vi "apply mapping changes.vi"(4 "original channel":refnum<class "TBM channel.lvclass">, 6 "original tag":string, 7 "owner ID":string, 8 "error in":errorcluster, 9 "channel":refnum<class "TBM channel.lvclass">, 10 "tag name":string, 11 "engine configuration in":refnum<class "engine configuration.lvclass">) -> (0 "error out":errorcluster, 3 "engine configuration out":refnum<class "engine configuration.lvclass">)   [LabVIEW 2014, in "engine configuration.lvclass"]
doc: "This function is meant as a catch-all for any changes in a channel or in a tag. The function will look at the original tag and original channel, compare that to the new tag and new channel, and take any steps necessary to update the engine configuration appropriately."
uses:
  engine configuration.lvclass
  <vilib>/NI/Tag Bus Module Framework/channel/TBM channel.lvclass
  <vilib>/NI/Tag Bus/tag/tag descriptor.lvclass/tag descriptor.ctl
  <vilib>/NI/Tag Bus Module Framework/channel/TBM channel.lvclass/TBM channel.ctl
  <vilib>/NI/Tag Bus/tag/tag descriptor.lvclass
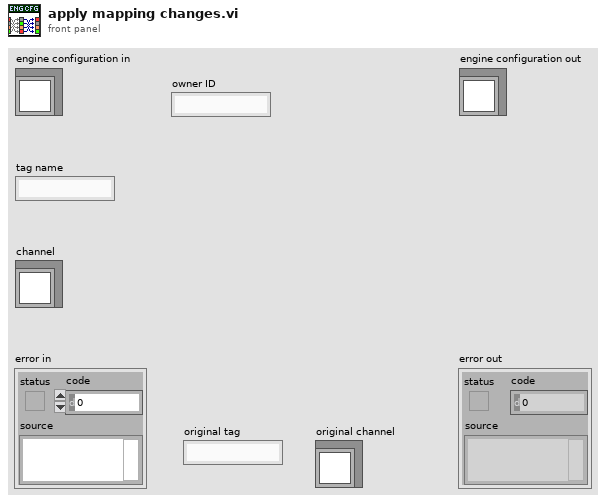
[diagram p1: front panel]
types:
  T1 = typedef "TBM channel.lvclass/channel classification.ctl" = enum16{"input data", "output data", "processing parameter", "processing result"}
  T2 = typedef "tag bus.lvlib/tag descriptor.lvclass/Data Type.ctl" = enum16{"Double", "Single", "I64", "I32", "I16", "I8", "U64", "U32", "U16", "U8", "Boolean", "String", "Array of Double", "Array of Single", "Array of I64", "Array of I32", "Array of I16", "Array of I8", "Array of U64", "Array of U32", "Array of U16", "Array of U8", "Array of Boolean", "Array of String"}
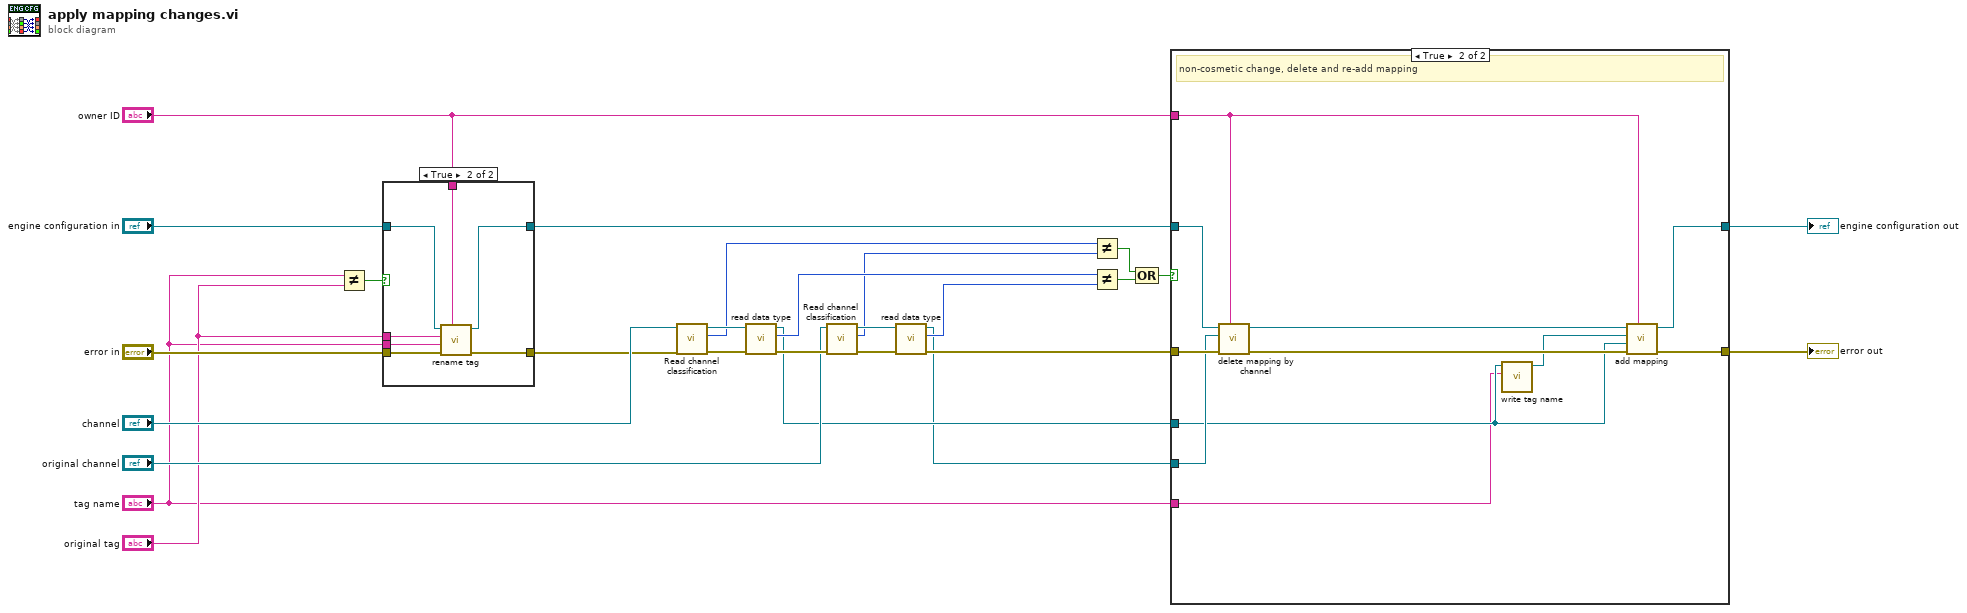
[diagram p0: block diagram]
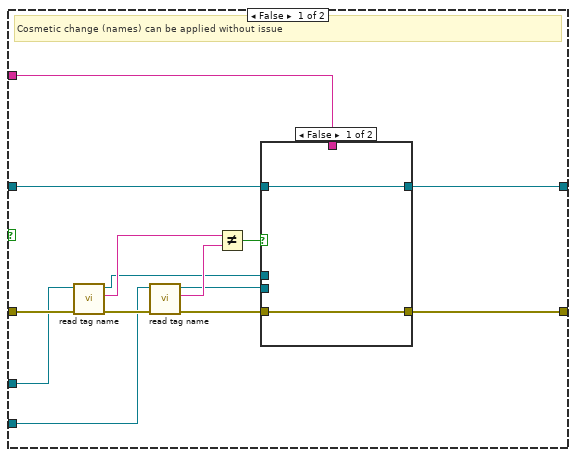
[diagram p3: hidden frame]
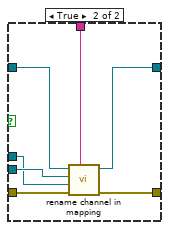
[diagram p4: hidden frame]
diagram:
  n1 = Not Equal?(x="tag name", y="original tag") -> (x != y?=w8:bool)
  n2 = case shown="True" w8 {
    tunnel: "error in" -> [w29 w36]
    tunnel: [w28 w34] -> w6
    tunnel: [w29 w35] -> w5
    tunnel: "engine configuration in" -> [w28 w33]
    tunnel: "owner ID" -> [_ w32]
    tunnel: "original tag" -> [_ w31]
    tunnel: "tag name" -> [_ w30]
    frame False {
    }
    frame True {
      n3 = call "rename tag.vi"("owner ID"=w32, "error in"=w36, "new name"=w30, "old name"=w31, "engine configuration in"=w33) -> ("error out"=w35:errorcluster, "engine configuration out"=w34:refnum<class "engine configuration.lvclass">)  [unwired: 5 in]
    }
  }
  n4 = call <vilib>:"Read channel classification.vi"("error in"=w5, "channel in"="channel") -> ("error out"=w25:errorcluster, "channel classification"=w14:T1, "channel out"=w26:refnum<class "TBM channel.lvclass">)  [unwired: 7 in]
  n5 = call <vilib>:"read data type.vi"("error in"=w25, "system tag in"=w26) -> ("error out"=w22:errorcluster, "data type"=w16:T2, "system tag out"=w12:refnum<class "TBM channel.lvclass">)  [unwired: 7 in]
  n6 = call <vilib>:"Read channel classification.vi"("error in"=w22, "channel in"="original channel") -> ("error out"=w24:errorcluster, "channel classification"=w15:T1, "channel out"=w23:refnum<class "TBM channel.lvclass">)  [unwired: 7 in]
  n7 = call <vilib>:"read data type.vi"("error in"=w24, "system tag in"=w23) -> ("error out"=w20:errorcluster, "data type"=w17:T2, "system tag out"=w11:refnum<class "TBM channel.lvclass">)  [unwired: 7 in]
  n8 = Not Equal?(x=w14, y=w15) -> (x != y?=w18:bool)
  n9 = Not Equal?(x=w16, y=w17) -> (x != y?=w19:bool)
  n10 = Compound Arithmetic op=OR(w18, w19) -> (w13:bool)
  n11 = case shown="True" w13 {
    tunnel: w20 -> [w41 w70]
    tunnel: w12 -> [w38 w61]
    tunnel: w11 -> [w37 w68]
    tunnel: w6 -> [w39 w69]
    tunnel: [w43 w65] -> w10
    tunnel: [w42 w64] -> w9
    tunnel: "owner ID" -> [w40 w63]
    tunnel: "tag name" -> [_ w60]
    frame False {
      # "Cosmetic change (names) can be applied without issue"
      n12 = call <vilib>:"read tag name.vi"("error in"=w41, "system tag in"=w38) -> ("error out"=w50:errorcluster, "name"=w48:string, "system tag out"=w44:refnum<class "TBM channel.lvclass">)  [unwired: 7 in]
      n13 = call <vilib>:"read tag name.vi"("error in"=w50, "system tag in"=w37) -> ("error out"=w47:errorcluster, "name"=w49:string, "system tag out"=w45:refnum<class "TBM channel.lvclass">)  [unwired: 7 in]
      n14 = Not Equal?(x=w48, y=w49) -> (x != y?=w46:bool)
      n15 = case shown="False" w46 {
        tunnel: w47 -> [w51 w59]
        tunnel: w39 -> [w52 w58]
        tunnel: w40 -> [_ w57]
        tunnel: w45 -> [_ w56]
        tunnel: w44 -> [_ w55]
        tunnel: [w52 w54] -> w42
        tunnel: [w51 w53] -> w43
        frame False {
        }
        frame True {
          n16 = call "rename channel in mapping.vi"("owner ID"=w57, "error in"=w59, "new channel"=w55, "old channel"=w56, "engine configuration in"=w58) -> ("error out"=w53:errorcluster, "engine configuration out"=w54:refnum<class "engine configuration.lvclass">)  [unwired: 5 in]
        }
      }
    }
    frame True {
      # "non-cosmetic change, delete and re-add mapping"
      n17 = call "delete mapping by channel.vi"("owner ID"=w63, "error in"=w70, "channel"=w68, "engine configuration in"=w69) -> ("error out"=w66:errorcluster, "engine configuration out"=w67:refnum<class "engine configuration.lvclass">)  [unwired: 6 in]
      n18 = call <vilib>:"write tag name.vi"("name"=w60, "system tag in"=w61) -> ("system tag out"=w62:refnum<class "TBM channel.lvclass">)  [unwired: 8 in, 1 out]
      n19 = call-dynamic "add mapping.vi"("owner ID"=w63, "error in"=w66, "channel"=w61, "tag descriptor"=w62, "engine configuration"=w67) -> ("error out"=w65:errorcluster, "engine configuration out"=w64:refnum<class "engine configuration.lvclass">)  [unwired: 5 in]
    }
  }
  "error out" <- w10
  "engine configuration out" <- w9
